vi "SUB_Random_freqHZ.vi"(3 "lower freq(HZ)":dbl) -> (1 "Output freq(HZ)":dbl)   [LabVIEW 2011]
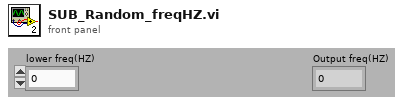
[diagram p1: front panel]
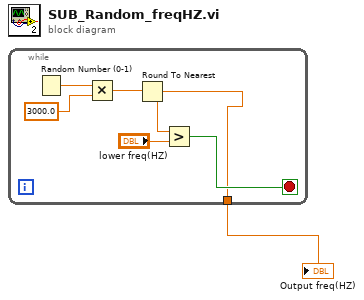
[diagram p0: block diagram]
diagram:
  n1 = while {
    tunnel: [w3] -> w1
    stop <- w4 stop-if-true
    n2 = Random Number (0-1)() -> (number: 0 to 1=w7:dbl)
    n3 = Multiply(x=w7, y=3000.0) -> (x*y=w5:dbl)
    n4 = Round To Nearest(number=w5) -> (nearest integer value=w3:dbl)
    n5 = Greater?(x=w3, y="lower freq(HZ)") -> (0:w4:bool)
  }
  "Output freq(HZ)" <- w1
